vi "FetchAddCorrection.vi"(0 "Azimuth Value":dbl, 1 "Vert Prof Array Index":u32, 3 "VP.TTHeightCorrs":T1={"Use Height Corrections"=TRUE, "TT.Azimuths"=[], "Z.HeightCorrs"=[], "Corrections from File"=TRUE, "Height Survey Filepaths"=[]}, 4 "Vert.Z-Locations":dbl[](array[numeric])=[12.7, 19.05, 25.4]) -> (5 "Vert.Z-Locations 2":dbl[](array[numeric])=[12.7, 19.05, 25.4], 6 "dz":dbl)   [LabVIEW 2015]
uses:
  CorrectionsCluster.ctl
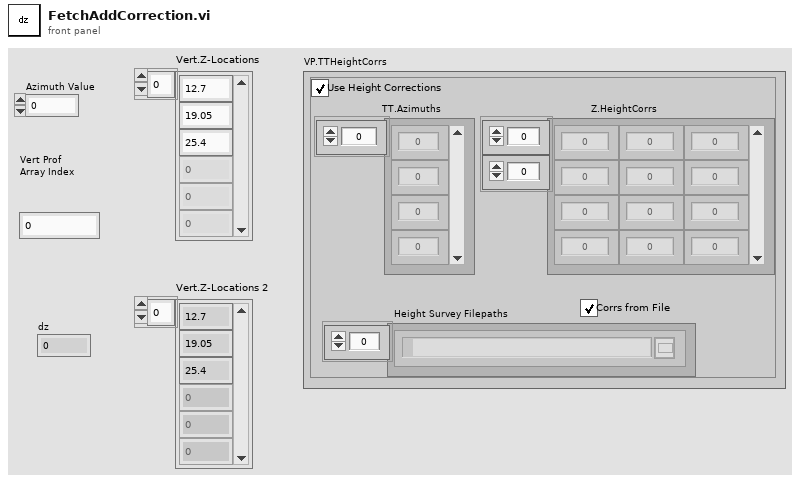
[diagram p1: front panel]
types:
  T1 = typedef "CorrectionsCluster.ctl" = cluster{"Use Height Corrections":bool, "TT.Azimuths":dbl[], "Z.HeightCorrs":dbl[][], "Corrections from File":bool, "Height Survey Filepaths":path[]}
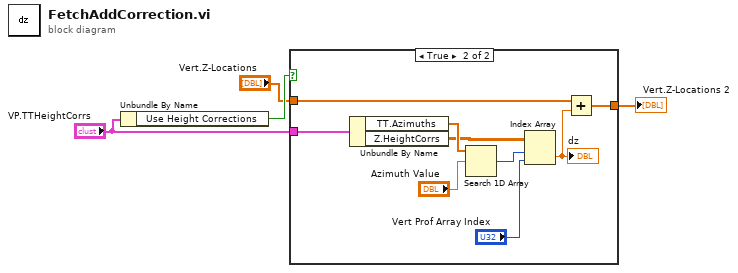
[diagram p0: block diagram]
diagram:
  n1 = Unbundle By Name("VP.TTHeightCorrs") -> ("Use Height Corrections"=w3:bool)
  n2 = case shown="True" w3 {
    tunnel: "VP.TTHeightCorrs" -> [_ w14]
    tunnel: [w5 w7] -> w1
    tunnel: "Vert.Z-Locations" -> [w5 w6]
    frame False {
    }
    frame True {
      n3 = Unbundle By Name(w14) -> ("TT.Azimuths"=w11:dbl[], "Z.HeightCorrs"=w9:dbl[][])
      n4 = Search 1D Array(1D array=w11, element="Azimuth Value") -> (index of element=w13:i32)  [unwired: 1 in]
      n5 = Index Array(array=w9, index (row)=w13, index (col)="Vert Prof Array Index") -> (element=w12:dbl)
      "dz" <- w12
      n6 = Add(x=w6, y=w12) -> (x+y=w7:dbl[])
    }
  }
  "Vert.Z-Locations 2" <- w1
